vi "N_Propiedades.vi"() -> ()   [LabVIEW 2021]
panel:
  in  "stop":bool
  # "Mendoza Meza Manuel Everardo"
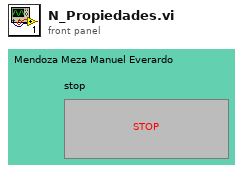
[diagram p1: front panel]
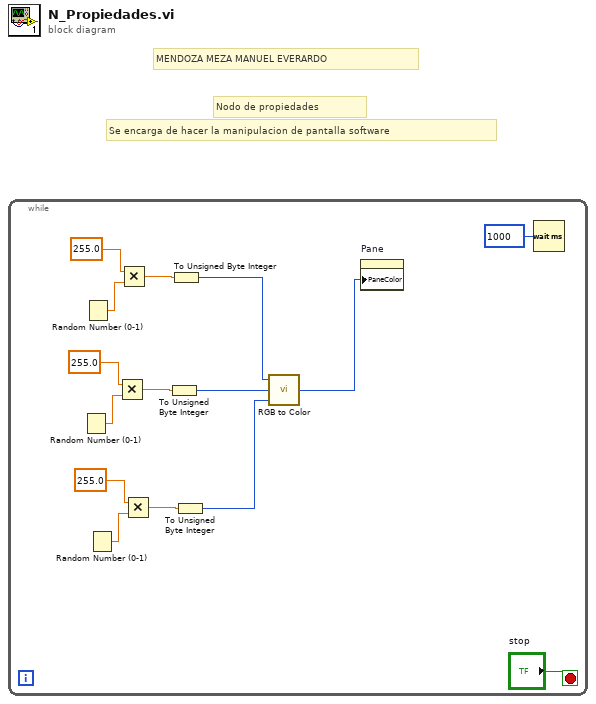
[diagram p0: block diagram]
diagram:
  # "MENDOZA MEZA MANUEL EVERARDO"
  # "Se encarga de hacer la manipulacion de pantalla software"
  # "Nodo de propiedades"
  n1 = while {
    stop <- "stop" stop-if-true
    n2 = Random Number (0-1)() -> (number: 0 to 1=w8:dbl)
    n3 = Random Number (0-1)() -> (number: 0 to 1=w13:dbl)
    n4 = Random Number (0-1)() -> (number: 0 to 1=w7:dbl)
    n5 = Multiply(x=255.0, y=w8) -> (x*y=w10:dbl)
    n6 = Multiply(x=255.0, y=w13) -> (x*y=w11:dbl)
    n7 = Multiply(x=255.0, y=w7) -> (x*y=w5:dbl)
    n8 = To Unsigned Byte Integer(number=w10) -> (unsigned 8bit integer=w3:u8)
    n9 = To Unsigned Byte Integer(number=w11) -> (unsigned 8bit integer=w4:u8)
    n10 = To Unsigned Byte Integer(number=w5) -> (unsigned 8bit integer=w2:u8)
    n11 = call <vilib>:"RGB to Color.vi"("B"=w2, "G"=w3, "R"=w4) -> ("Color"=w1:u32)
    n12 = property on="Pane" class="Pane"("PaneColor"=w1) -> ()  [unwired: 2 in, 2 out]
    n13 = Wait (ms)(milliseconds to wait=u32 1000) -> ()  [unwired: 1 out]
  }
